vi "test2.vi"() -> ()   [LabVIEW 2016]
uses:
  Electrometer/Electrometer.lvclass
  Electrometer/TempUnits.ctl
  ElectrometerConfiguration/ElectrometerConfiguration.lvclass
panel:
  out "Temperature":string
  out "READings":string
  out "error out":errorcluster
  in  "VISA":refnum<visa-resource-name>
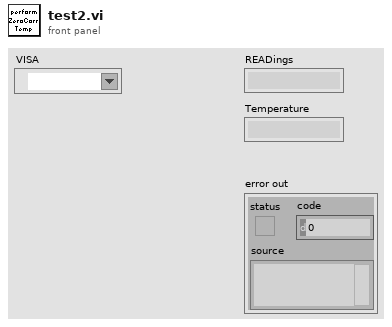
[diagram p1: front panel]
types:
  T1 = typedef "Electrometer.lvclass/TempUnits.ctl" = i32
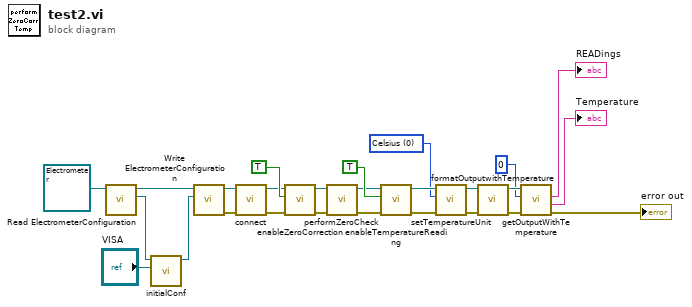
[diagram p0: block diagram]
diagram:
  w5 = T1 0 items=["Celsius", "Fahrenheit", "Kelvin"] ("Temperature Unit (0: Celsius)")
  n1 = call-dynamic "Read ElectrometerConfiguration.vi"("Electrometer in"=refnum<class "Electrometer.lvclass"> refnum ("Electrometer.lvclass")) -> ("ElectrometerConfiguration"=w25:refnum<class "ElectrometerConfiguration.lvclass">, "Electrometer out"=w22:refnum<class "Electrometer.lvclass">)  [unwired: 8 in, 1 out]
  n2 = call "initialConf.vi"("VISA"="VISA", "ElectrometerConfiguration In"=w25) -> ("ElectrometerConfiguration Out"=w23:refnum<class "ElectrometerConfiguration.lvclass">)  [unwired: 9 in]
  n3 = call-dynamic "Write ElectrometerConfiguration.vi"("ElectrometerConfiguration"=w23, "Electrometer in"=w22) -> ("error out"=w21:errorcluster, "Electrometer out"=w20:refnum<class "Electrometer.lvclass">)  [unwired: 8 in]
  n4 = call "connect.vi"("error in (no error)"=w21, "Electrometer in"=w20) -> ("error out"=w17:errorcluster, "Electrometer out"=w18:refnum<class "Electrometer.lvclass">)  [unwired: 7 in, 1 out]
  n5 = call "enableZeroCorrection.vi"("error in (no error)"=w17, "Enable Zero Check (T: Enable)"=TRUE, "Electrometer in"=w18) -> ("error out"=w16:errorcluster, "Electrometer out"=w15:refnum<class "Electrometer.lvclass">)  [unwired: 7 in]
  n6 = call "performZeroCheck.vi"("error in (no error)"=w16, "Electrometer in"=w15) -> ("error out"=w7:errorcluster, "Electrometer out"=w8:refnum<class "Electrometer.lvclass">)  [unwired: 8 in]
  n7 = call "enableTemperatureReading.vi"("error in (no error)"=w7, "Enable Temperature (T: Enable)"=TRUE, "Electrometer in"=w8) -> ("error out"=w4:errorcluster, "Electrometer out"=w6:refnum<class "Electrometer.lvclass">)  [unwired: 7 in]
  n8 = call "setTemperatureUnit.vi"("error in (no error)"=w4, "Temperature Unit (0: Celsius)"=w5, "Electrometer in"=w6) -> ("error out"=w2:errorcluster, "Electrometer out"=w3:refnum<class "Electrometer.lvclass">)  [unwired: 7 in]
  n9 = call "formatOutputwithTemperature.vi"("error in (no error)"=w2, "Electrometer in"=w3) -> ("error out"=w12:errorcluster, "Electrometer out"=w14:refnum<class "Electrometer.lvclass">)  [unwired: 8 in]
  n10 = call "getOutputWithTemperature.vi"("error in (no error)"=w12, "Reading Option (0: Latest)"=0, "Electrometer in"=w14) -> ("error out"=→"error out":errorcluster, "Temperature"=→"Temperature":string, "READings"=→"READings":string)  [unwired: 5 in, 1 out]
